vi "Modify NetworkObjects.vi"(0 "Connections":map{string, string}(c390)={"10.0.0.104"="norm"}, 2 "Command (list)":T1=enum."import", 11 "error in":errorcluster) -> (15 "error out":errorcluster)   [LabVIEW 2025]
uses:
  NetworkObjects Command.ctl
panel:
  in  "location":string="EvalLab"
  in  "host":string="10.0.0.156"
  in  "name":string="computername"
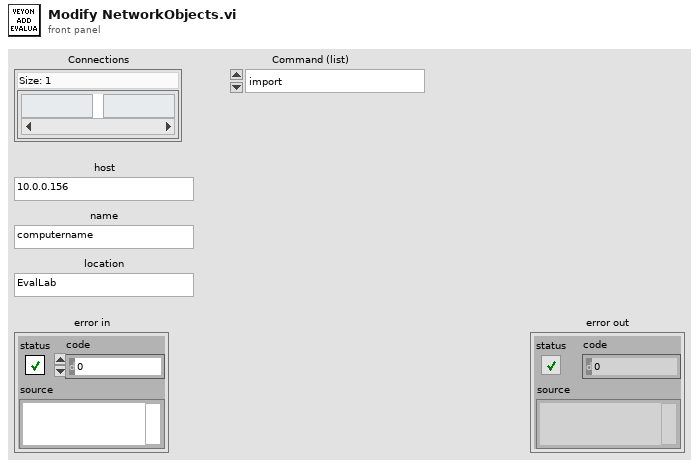
[diagram p1: front panel]
types:
  T1 = typedef "NetworkObjects Command.ctl" = enum16{"add computer", "add location", "clear", "dump", "export", "import", "list", "remove"}
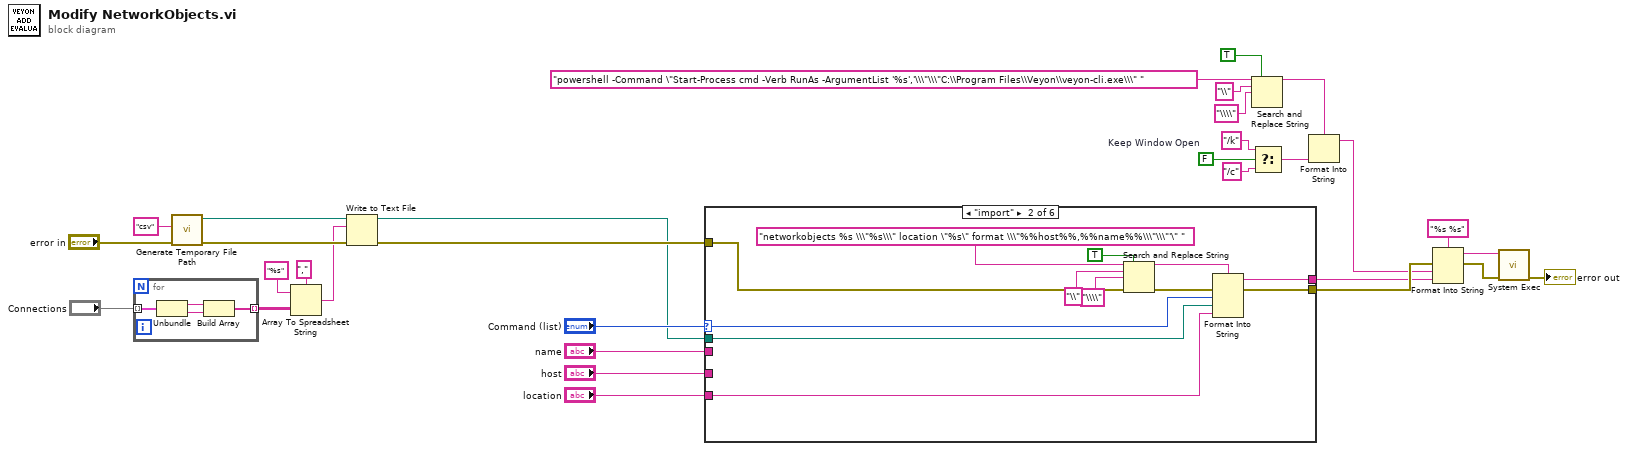
[diagram p0: block diagram]
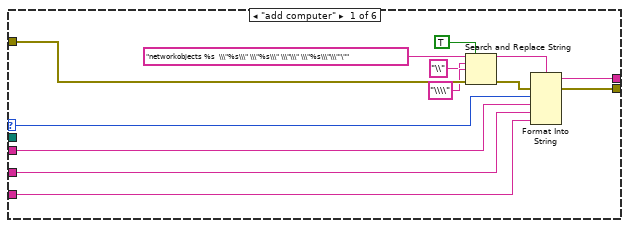
[diagram p2: hidden frame]
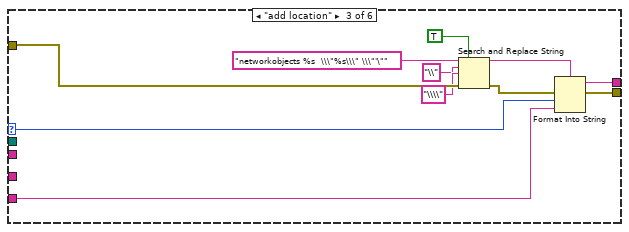
[diagram p3: hidden frame]
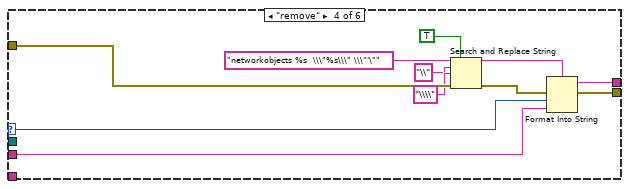
[diagram p4: hidden frame]
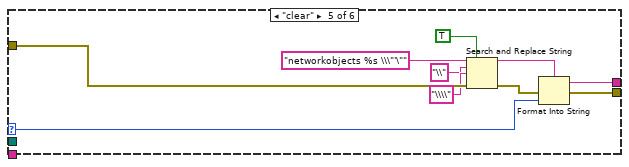
[diagram p5: hidden frame]
diagram:
  w22 = FALSE  # Keep Window Open
  n1 = for {
    tunnel: "Connections" -> [w34] mode=indexing
    tunnel: [w31] -> w7 mode=indexing
    n2 = Unbundle(w34) -> ("IP"=w33:string, "User ID"=w32:string)
    n3 = Build Array(w33, w32) -> (w31:string[])
  }
  n4 = call <vilib>:"Generate Temporary File Path.vi"("error in (no error)"="error in", "Temporary File Extension (tmp)"="csv") -> ("error out"=w29:errorcluster, "Unique Temporary File Path"=w2:path)  [unwired: 8 in]
  n5 = Array To Spreadsheet String(delimiter (Tab)=",", array=w7, 3:"%s" ("format string")) -> (spreadsheet string=w5:string)
  n6 = Write to Text File(file (use dialog)=w2, text=w5, error in=w29) -> (error out=w30:errorcluster)  [unwired: 1 in, 2 out]
  n7 = case shown="\"import\"" "Command (list)" {
    selector: "Command (list)" -> [w44 w53 w67 w78 w88 _]
    tunnel: "name" -> [w43 _ _ w71 _ _]
    tunnel: "host" -> [w42 _ _ _ _ _]
    tunnel: "location" -> [w41 w51 w60 _ _ _]
    tunnel: [w40 w50 w66 w77 w87 _] -> w15
    tunnel: w2 -> [_ w52 _ _ _ _]
    tunnel: w30 -> [w47 w59 w68 w81 w89 w92]
    tunnel: [w45 w57 w70 w79 w91 w92] -> w28
    frame "add computer" {
      n8 = Search and Replace String(replace all?=TRUE ("replace all? (F)"), input string="networkobjects %s  \\\"%s\\\" \\\"%s\\\" \\\"\\\" \\\"%s\\\"\\\"'\"", search string="\\", replace string="\\\\" ("replace string (\"\")"), error in=w47) -> (result string=w35:string, error out=w46:errorcluster)  [unwired: 3 in, 2 out]
      n9 = Format Into String(format string=w35, error in=w46, w44, w43, w42, w41) -> (resulting string=w40:string, error out=w45:errorcluster)  [unwired: 1 in]
    }
    frame "import" {
      n10 = Search and Replace String(replace all?=TRUE ("replace all? (F)"), input string="networkobjects %s \\\"%s\\\" location \"%s\" format \\\"%%host%%,%%name%%\\\"\\\"'\" ", search string="\\", replace string="\\\\" ("replace string (\"\")"), error in=w59) -> (result string=w54:string, error out=w58:errorcluster)  [unwired: 3 in, 2 out]
      n11 = Format Into String(format string=w54, error in=w58, w53, w52, w51) -> (resulting string=w50:string, error out=w57:errorcluster)  [unwired: 1 in]
    }
    frame "add location" {
      n12 = Search and Replace String(replace all?=TRUE ("replace all? (F)"), input string="networkobjects %s  \\\"%s\\\" \\\"'\"", search string="\\", replace string="\\\\" ("replace string (\"\")"), error in=w68) -> (result string=w61:string, error out=w69:errorcluster)  [unwired: 3 in, 2 out]
      n13 = Format Into String(format string=w61, error in=w69, w67, w60) -> (resulting string=w66:string, error out=w70:errorcluster)  [unwired: 1 in]
    }
    frame "remove" {
      n14 = Search and Replace String(replace all?=TRUE ("replace all? (F)"), input string="networkobjects %s  \\\"%s\\\" \\\"'\"", search string="\\", replace string="\\\\" ("replace string (\"\")"), error in=w81) -> (result string=w72:string, error out=w80:errorcluster)  [unwired: 3 in, 2 out]
      n15 = Format Into String(format string=w72, error in=w80, w78, w71) -> (resulting string=w77:string, error out=w79:errorcluster)  [unwired: 1 in]
    }
    frame "clear" {
      n16 = Search and Replace String(replace all?=TRUE ("replace all? (F)"), input string="networkobjects %s \\\"'\"", search string="\\", replace string="\\\\" ("replace string (\"\")"), error in=w89) -> (result string=w82:string, error out=w90:errorcluster)  [unwired: 3 in, 2 out]
      n17 = Format Into String(format string=w82, error in=w90, w88) -> (resulting string=w87:string, error out=w91:errorcluster)  [unwired: 1 in]
    }
    frame Default {
    }
  }
  n18 = Search and Replace String(replace all?=TRUE ("replace all? (F)"), input string="powershell -Command \"Start-Process cmd -Verb RunAs -ArgumentList '%s','\\\"\\\"C:\\Program Files\\Veyon\\veyon-cli.exe\\\" ", search string="\\", replace string="\\\\" ("replace string (\"\")")) -> (result string=w4:string)  [unwired: 4 in, 3 out]
  n19 = Select(t="/k", s=w22, f="/c") -> (s? t:f=w17:string)
  n20 = Format Into String(format string=w4, w17) -> (resulting string=w16:string)  [unwired: 2 in, 1 out]
  n21 = Format Into String(format string="%s %s", error in=w28, w16, w15) -> (resulting string=w10:string, error out=w27:errorcluster)  [unwired: 1 in]
  n22 = call <vilib>:"System Exec.vi"("error in (no error)"=w27, "command line"=w10) -> ("error out"=→"error out":errorcluster)  [unwired: 6 in, 3 out]
